vi "Force Close Window.vi"(8 "error in (no error)":errorcluster caption="错误输入（无错误）", 11 "User Interface 输入":refnum<class "User Interface.lvclass">) -> (0 "error out":errorcluster caption="错误输出", 3 "User Interface 输出":refnum<class "User Interface.lvclass">)   [LabVIEW 2018, in "MainInterface.lvlib" / "User Interface.lvclass"]
uses:
  User Interface.lvclass
  User Interface.lvclass/User Interface.ctl
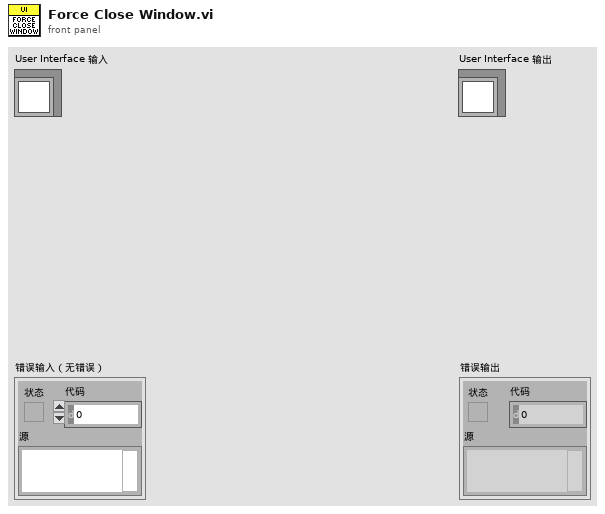
[diagram p1: front panel]
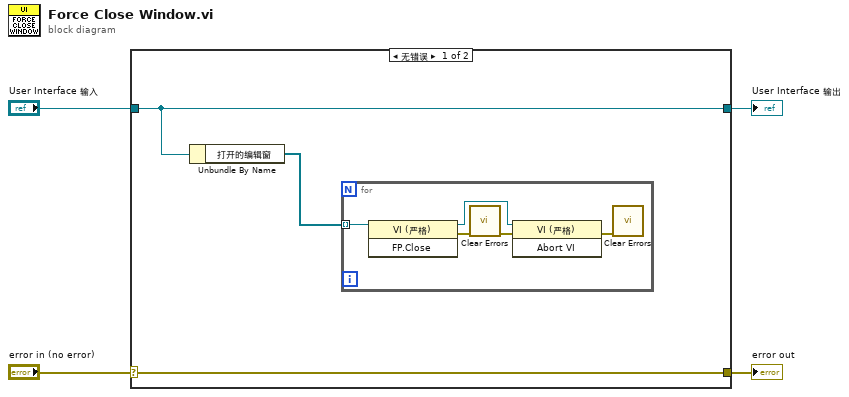
[diagram p0: block diagram]
diagram:
  n1 = case shown="无错误" "error in (no error)" {
    selector: "error in (no error)" -> [w7 w14]
    tunnel: [w7 w14] -> w3
    tunnel: [w6 w13] -> w1
    tunnel: "User Interface 输入" -> [w6 w13]
    frame No Error {
      n2 = Unbundle By Name(w6) -> ("打开的编辑窗"=w5:refnum<vi>[])
      n3 = for {
        tunnel: w5 -> [w12] mode=indexing
        n4 = invoke class="VI (严格)" method="FP.Close"(reference=w12) -> (reference out=w11:refnum<vi>, error out=w10:errorcluster)  [unwired: 2 in, 1 out]
        n5 = call <vilib>:"Clear Errors.vi"("error in (no error)"=w10) -> ("error out"=w9:errorcluster)  [unwired: 5 in, 1 out]
        n6 = invoke class="VI (严格)" method="Abort VI"(reference=w11, error in=w9) -> (error out=w8:errorcluster)  [unwired: 1 in, 2 out]
        n7 = call <vilib>:"Clear Errors.vi"("error in (no error)"=w8) -> ()  [unwired: 5 in, 2 out]
      }
    }
    frame Error {
    }
  }
  "error out" <- w3
  "User Interface 输出" <- w1
